vi "iconName.set.vi"(8 "error in (no error)":errorcluster, 10 "iconName":string, 11 "type in":refnum<class "type.lvclass">) -> (0 "error out":errorcluster, 3 "type out":refnum<class "type.lvclass">)   [LabVIEW 2020, in "type.lvclass"]
uses:
  type.lvclass
  type.lvclass/type.ctl
  Nominal Client/Nominal Client.lvclass
  3ddc10c0-dff5-4ae8-a87f-bac8ced954c2.vi
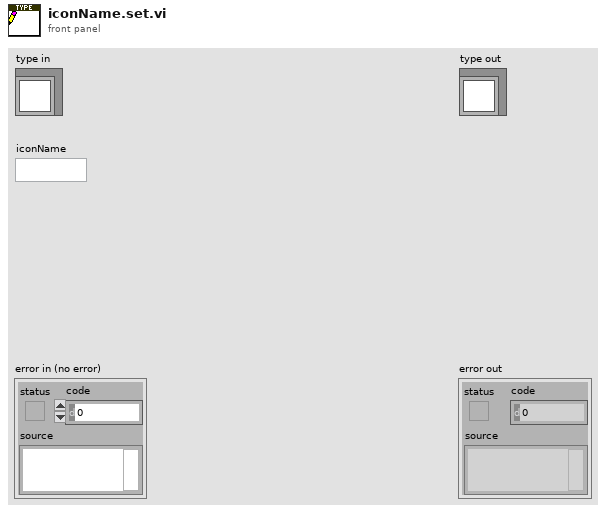
[diagram p1: front panel]
types:
  T1 = typedef "type.lvclass/typeData.ctl" = cluster{"rid":string, "name":string, "description":string, "propertyConfigs":T2, "createdAt":timestamp, "datasourceConfigs":T5[], "iconName":string}
  T2 = typedef "type.lvclass/properties.ctl" = T3[]
  T3 = typedef "type.lvclass/property.ctl" = cluster{"name":string, "value":T4}
  T4 = typedef "type.lvclass/property value.ctl" = cluster{"isRequired":bool, "description":string}
  T5 = typedef "type.lvclass/datasourceConfig.ctl" = cluster{"name":string, "v1":string[], "suggestedRefName":string}
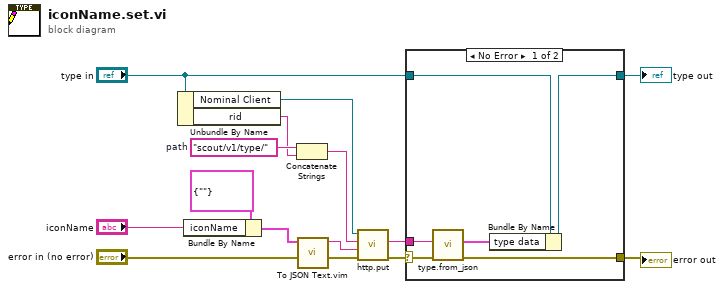
[diagram p0: block diagram]
diagram:
  w11 = "scout/v1/type/"  # path
  n1 = Unbundle By Name("type in") -> ("Nominal Client"=w15:refnum<class "Nominal Client.lvclass">, "rid"=w8:string)
  n2 = Bundle By Name(cluster=cluster{"iconName":string} {"iconName"=""}, "iconName"="iconName") -> (w13:cluster{"iconName":string})
  n3 = Concatenate Strings(w11, w8) -> (w10:string)
  n4 = call "To JSON Text.vim"("error in (no error)"="error in (no error)", "Anything"=w13) -> ("error out"=w9:errorcluster, "<JSON>"=w12:string)  [unwired: 8 in]
  n5 = call "http.put.vi"("error in"=w9, "Body"=w12, "Path"=w10, "Nominal Client in"=w15) -> ("error out"=w3:errorcluster, "Response"=w4:string)  [unwired: 4 in, 2 out]
  n6 = case shown="No Error" w3 {
    selector: w3 -> [w18 w23]
    tunnel: [w20 w23] -> w5
    tunnel: w4 -> [w19 _]
    tunnel: "type in" -> [w17 w22]
    tunnel: [w16 w22] -> w1
    frame No Error {
      n7 = call "type.from_json.vi"("error in"=w18, "json"=w19) -> ("error out"=w20:errorcluster, "type data"=w21:T1)  [unwired: 8 in]
      n8 = Bundle By Name(cluster=w17, "type data"=w21) -> (w16:refnum<class "type.lvclass">)
    }
    frame Error {
    }
  }
  "error out" <- w5
  "type out" <- w1
